vi "DTC_ERASE.vi"(8 "errin":errorcluster, 11 "UNINIT?":bool) -> (0 "error out":errorcluster, 3 "Erased?":bool)   [LabVIEW 2020]
uses:
  <userlib>/PCAN Basic/Controls/BaudrateEenum.ctl
  <userlib>/PCAN Basic/Controls/Channel.ctl
  c81b2dea-558f-4924-9439-a6ac718f321b.vi
  c8c4598e-5b6f-4378-8c15-02bdfed9a775.vi
  9d8e4623-a32b-447d-80bb-b40a32a310c5.vi
  OP500/VG/VG_branche.vi
  <userlib>/Alex_Peak_lib/PEAK_lib_ALEX.lvlib
  <userlib>/PCAN Basic/PCANBasic.lvlib
panel:
  out "101":u8[](array[numeric])
  out "dataout":T1
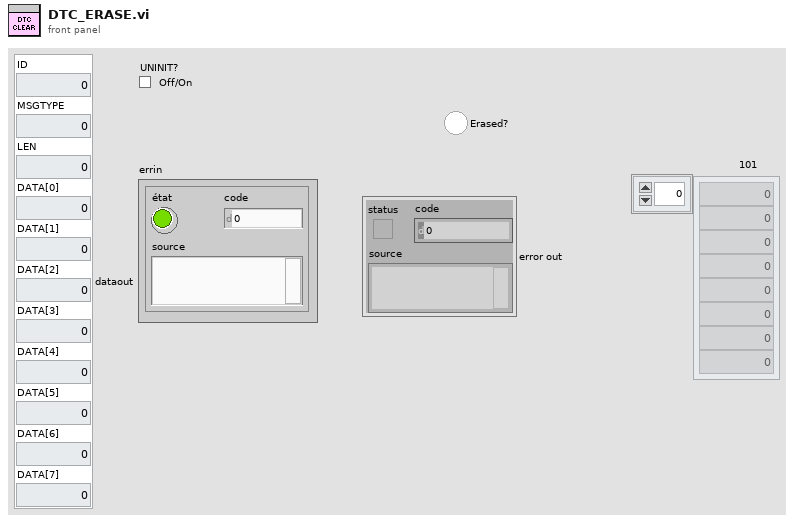
[diagram p1: front panel]
types:
  T1 = cluster{"ID":u32, "MSGTYPE":u8, "LEN":u8, "DATA[0]":u8, "DATA[1]":u8, "DATA[2]":u8, "DATA[3]":u8, "DATA[4]":u8, "DATA[5]":u8, "DATA[6]":u8, "DATA[7]":u8}
  T2 = typedef "PCANBasic.lvlib/Channel.ctl" = enum16{"PCAN_NONEBUS", "not used1", "not used2", "not used3", "not used4", "not used5", "not used6", "not used7", "not used8", "not used9", "not used10", "not used11", "not used12", "not used13", "not used14", "not used15", "not used16", "not used17", "not used18", "not used19", "not used20", "not used21", "not used22", "not used23", "not used24", "not used25", "not used26", "not used27", "not used28", "not used29", "not used30", "not used31", "not used32", "PCAN_ISABUS1", "PCAN_ISABUS2", "PCAN_ISABUS3", "PCAN_ISABUS4", "PCAN_ISABUS5", "PCAN_ISABUS6", "PCAN_ISABUS7", "PCAN_ISABUS8", "not used41", "not used42", "not used43", "not used44", "not used45", "not used46", "not used47", "not used48", "PCAN_DNGBUS1", "not used50", "not used51", "not used52", "not used53", "not used54", "not used55", "not used56", "not used57", "not used58", "not used59", "not used60", "not used61", "not used62", "not used63", "not used64", "PCAN_PCIBUS1", "PCAN_PCIBUS2", "PCAN_PCIBUS3", "PCAN_PCIBUS4", "PCAN_PCIBUS5", "PCAN_PCIBUS6", "PCAN_PCIBUS7", "PCAN_PCIBUS8", "not used73", "not used74", "not used75", "not used76", "not used77", "not used78", "not used79", "not used80", "PCAN_USBBUS1", "PCAN_USBBUS2", "PCAN_USBBUS3", "PCAN_USBBUS4", "PCAN_USBBUS5", "PCAN_USBBUS6", "PCAN_USBBUS7", "PCAN_USBBUS8", "Not used89", "Not used90", "Not used91", "Not used92", "Not used93", "Not used94", "Not used95", "Not used96", "PCAN_PCCBUS1", "PCAN_PCCBUS2"}
  T3 = typedef "PCANBasic.lvlib/BaudrateEenum.ctl" = enum16{"CAN_Baud_1M", "CAN_Baud_800K", "CAN_BAUD_500K", "CAN_BAUD_250K", "CAN_BAUD_125K", "CAN_BAUD_100K", "CAN_BAUD_95K", "CAN_BAUD_83K", "CAN_BAUD_50K", "CAN_BAUD_47K", "CAN_BAUD_33K", "CAN_BAUD_20K", "CAN_BAUD_10K", "CAN_BAUD_5K", "User Baudrate"}
  T4 = cluster{"ID":u32, "MSGTYPE":u8, "LEN":u8, "DATA[0]":ext, "DATA[1]":ext, "DATA[2]":ext, "DATA[3]":ext, "DATA[4]":ext, "DATA[5]":ext, "DATA[6]":ext, "DATA[7]":ext}
  T5 = cluster{"DATA[0]":ext, "DATA[1]":ext, "DATA[2]":ext, "DATA[3]":ext, "DATA[4]":ext, "DATA[5]":ext, "DATA[6]":ext, "DATA[7]":ext}
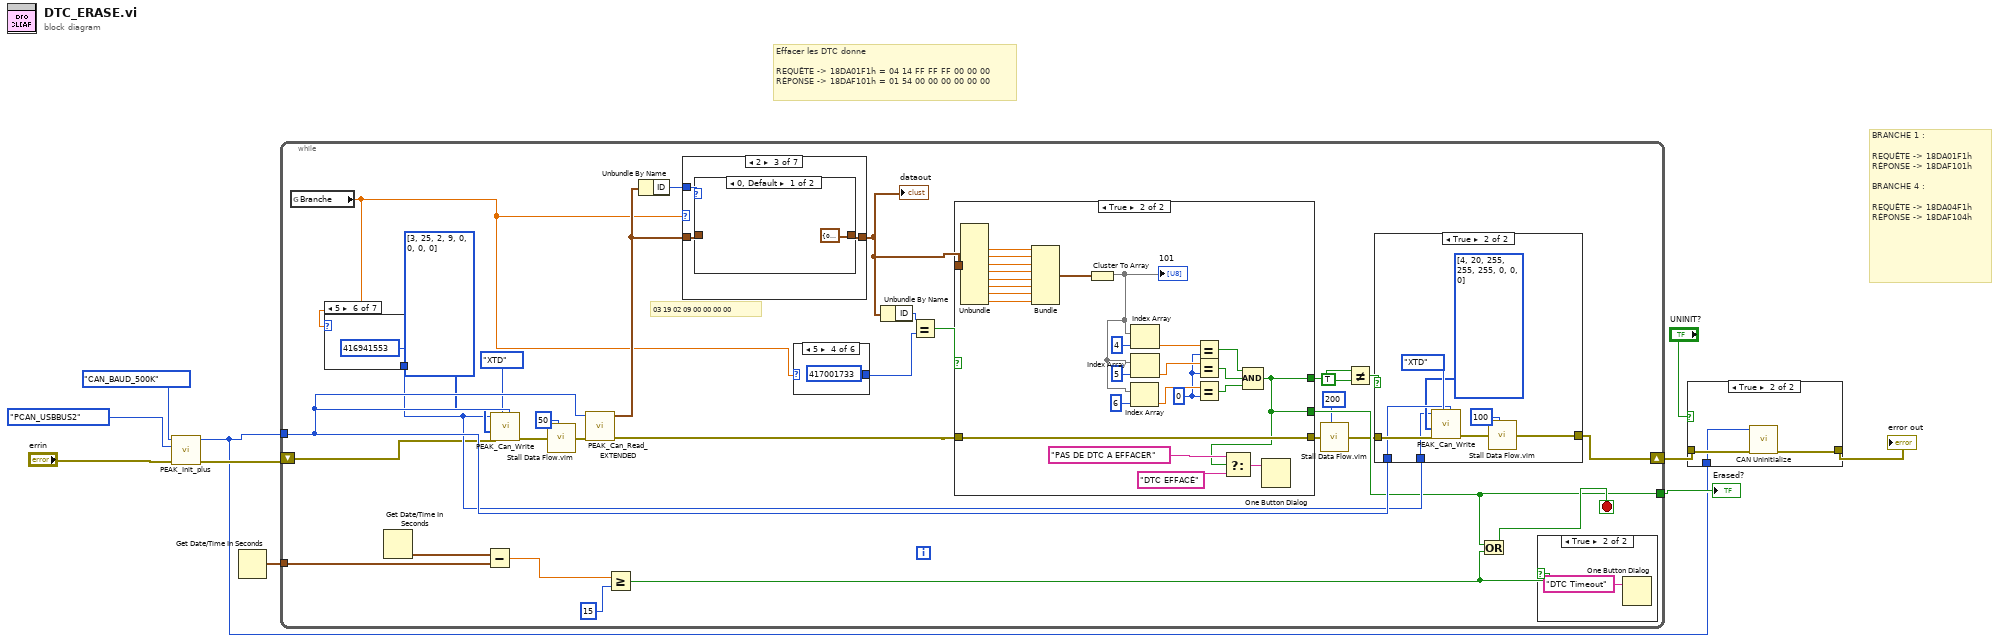
[diagram p0: block diagram]
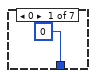
[diagram p4: hidden frame]
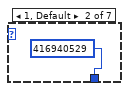
[diagram p5: hidden frame]
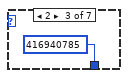
[diagram p6: hidden frame]
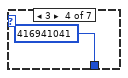
[diagram p7: hidden frame]
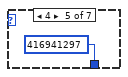
[diagram p8: hidden frame]
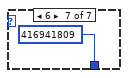
[diagram p9: hidden frame]
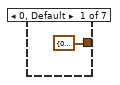
[diagram p10: hidden frame]
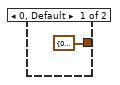
[diagram p12: hidden frame]
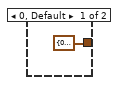
[diagram p15: hidden frame]
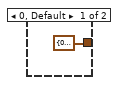
[diagram p17: hidden frame]
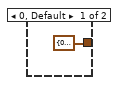
[diagram p19: hidden frame]
diagram:
  # "BRANCHE 1 :\n\nREQUÊTE -> 18DA01F1h\nRÉPONSE -> 18DAF101h\n\nBRANCHE 4 :\n\nREQUÊTE -> 18DA04F1h\nRÉPONSE -> 18DAF104h"
  # "Effacer les DTC donne \n\nREQUÊTE -> 18DA01F1h = 04 14 FF FF FF 00 00 00\nRÉPONSE -> 18DAF101h = 01 54 00 00 00 00 00 00"
  n1 = call <userlib>:"PEAK_Init_plus.vi"("errin"="errin", "Channel"=Channel."PCAN_USBBUS2", "BTR0BTR1"=BaudrateEenum."CAN_BAUD_500K") -> ("errout"=w10:errorcluster, "Channel out"=w1:T2)  [unwired: 7 in]
  n2 = Get Date/Time In Seconds() -> (seconds since 1Jan1904=w7:timestamp)
  n3 = while {
    tunnel: w1 -> [w35]
    shift-right: [w24] -> w6
    shift-left: w10 -> [w21]
    tunnel: [w19] -> w8
    tunnel: w7 -> [w18]
    stop <- w20 stop-if-true
    # "03 19 02 09 00 00 00 00"
    n4 = global read "VG_branche.vi" "Branche"() -> (w22:dbl)
    n5 = case shown="5" w22 {
      tunnel: [u32 0 ("Identifier") u32 416940529 ("Identifier") u32 416940785 ("Identifier") u32 416941041 ("Identifier") u32 416941297 ("Identifier") u32 416941553 ("Identifier") u32 416941809 ("Identifier")] -> w25
      frame 0 {
      }
      frame 1, Default {
      }
      frame 2 {
      }
      frame 3 {
      }
      frame 4 {
      }
      frame 5 {
      }
      frame 6 {
      }
    }
    n6 = Get Date/Time In Seconds() -> (seconds since 1Jan1904=w17:timestamp)
    n7 = Subtract(x=w17, y=w18) -> (x-y=w16:dbl)
    n8 = call <userlib>:"PEAK_Can_Write.vi"("CAN handle"=w35, "MSG type"=enum8{"STD", "RTR", "XTD", "XTD RTR", "STATUS"}."XTD", "errin"=w21, "CAN Data"=i32[] [3, 25, 2, 9, 0, 0, 0, 0], "Identifier"=w25) -> ("errout"=w31:errorcluster)  [unwired: 6 in]
    n9 = call "Stall Data Flow.vim"("value in"=w31, "milliseconds to wait"=u32 50) -> ("value out"=w29:errorcluster)  [unwired: 1 out]
    n10 = call <userlib>:"PEAK_Can_Read_EXTENDED.vi"("errin"=w29, "Channel out"=w35) -> ("errout"=w39:errorcluster, "MessageBuffer out"=w33:T4)  [unwired: 7 in, 1 out]
    n11 = Greater Or Equal?(x=w16, y=15) -> (x >= y?=w14:bool)
    n12 = Unbundle By Name(w33) -> ("ID"=w34:u32)
    n13 = case shown="2" w22 {
      tunnel: w34 -> [_ w60 w65 w70 w75 w80 w84]
      tunnel: w33 -> [_ w59 w64 w69 w74 w79 w85]
      tunnel: [T1 {"ID"=0, "MSGTYPE"=0, "LEN"=0, "DATA[0]"=0, "DATA[1]"=0, "DATA[2]"=0, "DATA[3]"=0, "DATA[4]"=0, "DATA[5]"=0, "DATA[6]"=0, "DATA[7]"=0} ("MessageBuffer out") w58 w63 w68 w73 w78 w83] -> w40
      frame 0, Default {
      }
      frame 1 {
        # "Fonction branche"
        n14 = case shown="18DAF101" w60 {
          tunnel: w59 -> [_ w62]
          tunnel: [T1 {"ID"=0, "MSGTYPE"=0, "LEN"=0, "DATA[0]"=0, "DATA[1]"=0, "DATA[2]"=0, "DATA[3]"=0, "DATA[4]"=0, "DATA[5]"=0, "DATA[6]"=0, "DATA[7]"=0} ("MessageBuffer out") w62] -> w58
          frame 0, Default {
          }
          frame 417001729 {
          }
        }
      }
      frame 2 {
        n15 = case shown="0, Default" w65 {
          tunnel: w64 -> [_ w67]
          tunnel: [T1 {"ID"=0, "MSGTYPE"=0, "LEN"=0, "DATA[0]"=0, "DATA[1]"=0, "DATA[2]"=0, "DATA[3]"=0, "DATA[4]"=0, "DATA[5]"=0, "DATA[6]"=0, "DATA[7]"=0} ("MessageBuffer out") w67] -> w63
          frame 0, Default {
          }
          frame 417001730 {
          }
        }
      }
      frame 3 {
        n16 = case shown="18DAF103" w70 {
          tunnel: w69 -> [_ w72]
          tunnel: [T1 {"ID"=0, "MSGTYPE"=0, "LEN"=0, "DATA[0]"=0, "DATA[1]"=0, "DATA[2]"=0, "DATA[3]"=0, "DATA[4]"=0, "DATA[5]"=0, "DATA[6]"=0, "DATA[7]"=0} ("MessageBuffer out") w72] -> w68
          frame 0, Default {
          }
          frame 417001731 {
          }
        }
      }
      frame 4 {
        n17 = case shown="18DAF104" w75 {
          tunnel: w74 -> [_ w77]
          tunnel: [T1 {"ID"=0, "MSGTYPE"=0, "LEN"=0, "DATA[0]"=0, "DATA[1]"=0, "DATA[2]"=0, "DATA[3]"=0, "DATA[4]"=0, "DATA[5]"=0, "DATA[6]"=0, "DATA[7]"=0} ("MessageBuffer out") w77] -> w73
          frame 0, Default {
          }
          frame 417001732 {
          }
        }
      }
      frame 5 {
        n18 = case shown="18DAF105" w80 {
          tunnel: w79 -> [_ w82]
          tunnel: [T1 {"ID"=0, "MSGTYPE"=0, "LEN"=0, "DATA[0]"=0, "DATA[1]"=0, "DATA[2]"=0, "DATA[3]"=0, "DATA[4]"=0, "DATA[5]"=0, "DATA[6]"=0, "DATA[7]"=0} ("MessageBuffer out") w82] -> w78
          frame 0, Default {
          }
          frame 417001733 {
          }
        }
      }
      frame 6 {
        n19 = case shown="18DAF106" w84 {
          tunnel: [T1 {"ID"=0, "MSGTYPE"=0, "LEN"=0, "DATA[0]"=0, "DATA[1]"=0, "DATA[2]"=0, "DATA[3]"=0, "DATA[4]"=0, "DATA[5]"=0, "DATA[6]"=0, "DATA[7]"=0} ("MessageBuffer out") w87] -> w83
          tunnel: w85 -> [_ w87]
          frame 0, Default {
          }
          frame 417001734 {
          }
        }
      }
    }
    "dataout" <- w40
    n20 = case shown="5" w22 {
      tunnel: [417001730 417001731 417001732 417001733 417001734 417001729] -> w26
      frame 2 {
      }
      frame 3 {
      }
      frame 4 {
      }
      frame 5 {
      }
      frame 6 {
      }
      frame 1, Default {
      }
    }
    n21 = Unbundle By Name(w40) -> ("ID"=w27:u32)
    n22 = Equal?(x=w27, y=w26) -> (x = y?=w38:bool)
    n23 = case shown="True" w38 {
      tunnel: w40 -> [_ w112]
      tunnel: [w94 w98] -> w37
      tunnel: [w95 w99] -> w36
      tunnel: w39 -> [w95 w99]
      tunnel: [w94 w98] -> w19
      frame False {
        w94 = FALSE
      }
      frame True {
        w104 = u8 0 ("y")
        n24 = Unbundle(w112) -> ("DATA[0]"=w121:ext, "DATA[1]"=w120:ext, "DATA[2]"=w119:ext, "DATA[3]"=w118:ext, "DATA[4]"=w117:ext, "DATA[5]"=w116:ext, "DATA[6]"=w115:ext, "DATA[7]"=w114:ext)  [unwired: 3 out]
        n25 = Bundle("DATA[0]"=w121, "DATA[1]"=w120, "DATA[2]"=w119, "DATA[3]"=w118, "DATA[4]"=w117, "DATA[5]"=w116, "DATA[6]"=w115, "DATA[7]"=w114) -> (w113:T5)  [unwired: 1 in]
        n26 = Cluster To Array(cluster=w113) -> (array=w108:ext[])
        "101" <- w108
        n27 = Index Array(array=w108, index=6) -> (element=w105:ext)
        n28 = Index Array(array=w108, index=4) -> (element=w107:ext)
        n29 = Index Array(array=w108, index=5) -> (element=w106:ext)
        n30 = Equal?(x=w107, y=w104) -> (x = y?=w103:bool)
        n31 = Equal?(x=w106, y=w104) -> (x = y?=w102:bool)
        n32 = Equal?(x=w105, y=w104) -> (x = y?=w101:bool)
        n33 = Compound Arithmetic op=AND(w103, w102, w101) -> (w98:bool)
        n34 = Select(t="PAS DE DTC A EFFACER", s=w98, f="DTC EFFACÉ") -> (s? t:f=w96:string)
        n35 = One Button Dialog(message=w96) -> ()  [unwired: 1 in, 1 out]
      }
    }
    n36 = call "Stall Data Flow.vim"("value in"=w36, "milliseconds to wait"=u32 200) -> ("value out"=w13:errorcluster)  [unwired: 1 out]
    n37 = Not Equal?(x=w37, y=TRUE) -> (x != y?=w11:bool)
    n38 = case shown="True" w11 {
      tunnel: w13 -> [w41 w46]
      tunnel: w35 -> [_ w45]
      tunnel: w25 -> [_ w43]
      tunnel: [w41 w42] -> w24
      frame False {
      }
      frame True {
        n39 = call <userlib>:"PEAK_Can_Write.vi"("CAN handle"=w45, "MSG type"=enum8{"STD", "RTR", "XTD", "XTD RTR", "STATUS"}."XTD", "errin"=w46, "CAN Data"=i32[] [4, 20, 255, 255, 255, 0, 0, 0], "Identifier"=w43) -> ("errout"=w48:errorcluster)  [unwired: 6 in]
        n40 = call "Stall Data Flow.vim"("value in"=w48, "milliseconds to wait"=u32 100) -> ("value out"=w42:errorcluster)  [unwired: 1 out]
      }
    }
    n41 = Or(x=w19, y=w14) -> (x .or. y?=w20:bool)
    n42 = case shown="True" w14 {
      frame False {
      }
      frame True {
        n43 = One Button Dialog(message="DTC Timeout") -> ()  [unwired: 1 in, 1 out]
      }
    }
  }
  "Erased?" <- w8
  n44 = case shown="True" "UNINIT?" {
    tunnel: w6 -> [w123 w126]
    tunnel: [w123 w125] -> w5
    tunnel: w1 -> [_ w124]
    frame False {
    }
    frame True {
      n45 = call <userlib>:"CAN Uninitialize.vi"("error in (no error)"=w126, "Channel"=w124) -> ("error out"=w125:errorcluster)  [unwired: 7 in, 2 out]
    }
  }
  "error out" <- w5
